vi "Plug_in_BMT_data.vi"() -> (5 "Plug in titles":string[](array[string])=["Raw data filename", "A Left", "B Left", "A Right", "B Right", "Left Bkgd", "Right Bkgd", "Left C", "Right C", "Left c'/C", "Right c'/C"], 7 "Plug in values":string[](array[string])=["18-3-99_69", "-0.030963", "0.003450", "-0.009121", "0.004121", "10.850", "6.000", "36.577", "23.514", "1.502", "1.091"])   [LabVIEW 2010]
uses:
  Globals/Meas_global.vi
  Globals/Plug_in_data_global.vi
  <vilib>/Analysis/3filter.llb/Butterworth Filter (DBL).vi
  <vilib>/Analysis/NI_AALBase.lvlib
  <vilib>/Analysis/NI_AALPro.lvlib
panel:
  in  "Smooth":bool=TRUE
  in  "Filter":bool
  out "PDF Right":cluster{"Axis":dbl[], dbl[]}(graph)={"Axis"=[-35.0, -30.0, -25.0, -20.0, -15.0, -10.0, -5.0, 0.0, 5.0, 10.0, 15.0, 20.0, 25.0, 30.0, 35.0, 40.0, 45.0, 50.0, 55.0, 60.0, 65.0, 70.0, 75.0, 80.0, 85.0, 90.0, 95.0, 100.0, 105.0, 110.0, 115.0, 120.0, 125.0, 130.0, 135.0, 140.0, 145.0, 150.0, 155.0, 160.0, 165.0, 170.0, 175.0, 180.0, 185.0, 190.0, 195.0, 200.0, 205.0, 210.0, 215.0, 220.0, 225.0, 230.0, 235.0, 240.0, 245.0, 250.0, 255.0, 260.0, 265.0, 270.0, 275.0, 280.0, 285.0, 290.0, 295.0, 300.0, 305.0, 310.0, 315.0, 320.0, 325.0, 330.0, 335.0, 340.0, 345.0, 350.0, 355.0, 360.0, 365.0, 370.0, 375.0, 380.0, 385.0, 390.0, 395.0, 400.0, 405.0, 410.0, 415.0, 420.0, 425.0, 430.0, 435.0, 440.0, 445.0, 450.0, 455.0, 460.0, 465.0, 470.0, 475.0, 480.0, 485.0, 490.0, 495.0, 500.0], [0.0, 0.0, 0.0, 6.25e-05, 0.0001875, 0.0024375, 0.0111875, 0.090375, 0.154625, 0.15925, 0.1253125, 0.0861875, 0.074625, 0.0625, 0.0445, 0.03575, 0.0279375, 0.0205, 0.0174375, 0.0135625, 0.0113125, 0.0090625, 0.0081875, 0.006625, 0.0050625, 0.005, 0.0049375, 0.003625, 0.003625, 0.003125, 0.002, 0.002375, 0.0014375, 0.0009375, 0.00125, 0.000625, 0.0005, 0.000125, 0.0005625, 0.000375, 0.000375, 0.0001875, 0.00025, 0.0003125, 0.0001875, 0.00025, 0.00025, 0.00025, 0.000125, 6.25e-05, 0.0, 0.0001875, 6.25e-05, 6.25e-05, 0.0, 0.0, 0.0, 0.0, 0.000125, 0.0, 0.0, 0.0, 0.0, 6.25e-05, 0.0, 0.0, 0.0, 0.0, 0.0, 0.0, 0.0, 0.0, 0.0, 0.0, 0.0, 0.0, 0.0, 0.0, 0.0, 0.0, 0.0, 0.0, 0.0, 0.0, 0.0, 0.0, 0.0, 0.0, 0.0, 0.0, 0.0, 0.0, 0.0, 0.0, 0.0, 0.0, 0.0, 0.0, 0.0, 0.0, 0.0, 0.0, 0.0, 6.25e-05, 0.0, 0.0, 0.0, 0.0]}
  out "PDF Left":cluster{"Axis":dbl[], dbl[]}(graph)={"Axis"=[-35.0, -30.0, -25.0, -20.0, -15.0, -10.0, -5.0, 0.0, 5.0, 10.0, 15.0, 20.0, 25.0, 30.0, 35.0, 40.0, 45.0, 50.0, 55.0, 60.0, 65.0, 70.0, 75.0, 80.0, 85.0, 90.0, 95.0, 100.0, 105.0, 110.0, 115.0, 120.0, 125.0, 130.0, 135.0, 140.0, 145.0, 150.0, 155.0, 160.0, 165.0, 170.0, 175.0, 180.0, 185.0, 190.0, 195.0, 200.0, 205.0, 210.0, 215.0, 220.0, 225.0, 230.0, 235.0, 240.0, 245.0, 250.0, 255.0, 260.0, 265.0, 270.0, 275.0, 280.0, 285.0, 290.0, 295.0, 300.0, 305.0, 310.0, 315.0, 320.0, 325.0, 330.0, 335.0, 340.0, 345.0, 350.0, 355.0, 360.0, 365.0, 370.0, 375.0, 380.0, 385.0, 390.0, 395.0, 400.0, 405.0, 410.0, 415.0, 420.0, 425.0, 430.0, 435.0, 440.0, 445.0, 450.0, 455.0, 460.0, 465.0, 470.0, 475.0, 480.0, 485.0, 490.0, 495.0, 500.0], [0.0001875, 0.00025, 0.0003125, 0.000625, 0.00225, 0.0058125, 0.0179375, 0.1063125, 0.1238125, 0.1006875, 0.0925, 0.074875, 0.0638125, 0.05425, 0.045875, 0.0419375, 0.03625, 0.02475, 0.022625, 0.02125, 0.0186875, 0.0146875, 0.013625, 0.0095, 0.0085625, 0.0083125, 0.0081875, 0.007, 0.0065625, 0.00575, 0.0041875, 0.004875, 0.0043125, 0.0045, 0.003, 0.003375, 0.003, 0.0019375, 0.002625, 0.0025625, 0.001875, 0.0015, 0.0015, 0.0015625, 0.001625, 0.0011875, 0.00125, 0.0013125, 0.0011875, 0.0005625, 0.00075, 0.00075, 0.000875, 0.0006875, 0.0003125, 0.00075, 0.0003125, 0.0005625, 0.0003125, 0.0003125, 0.000375, 0.0005625, 0.0003125, 0.000375, 0.00025, 0.00025, 0.0005625, 0.00025, 0.0001875, 0.000375, 0.0003125, 0.0003125, 0.000125, 0.000125, 0.0001875, 6.25e-05, 0.0001875, 0.000125, 0.0, 6.25e-05, 0.0001875, 0.00025, 0.000125, 0.00025, 0.000125, 6.25e-05, 0.000125, 0.000125, 0.0, 0.000125, 6.25e-05, 0.000125, 6.25e-05, 0.0001875, 0.000125, 0.000125, 6.25e-05, 6.25e-05, 0.00025, 0.0, 6.25e-05, 0.0, 0.0, 0.0, 6.25e-05, 0.0, 6.25e-05, 0.000125]}
  in  "No of bins":i32=108
  in  "Min value":dbl=-37.5 format="%.2f"
  in  "Max value":dbl=502.5 format="%.2f"
  out "Right Bkgd ppm":dbl=6.0 format="%.2f"
  out "Left Bkgd ppm":dbl=10.85 format="%.2f"
  out "Right FID Smoothed data":T1(graph)
  out "Total time":dbl=159.92000000000004 format="%.2f"
  out "Left FID Smoothed data":T1(graph)
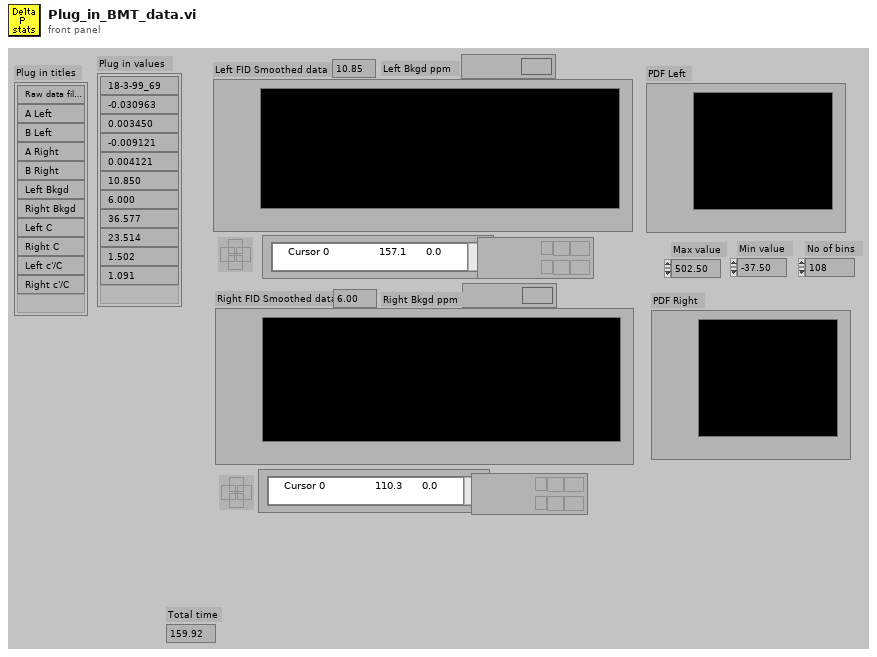
[diagram p1: front panel]
types:
  T1 = cluster{"X array Out":dbl[], "Y array Out":dbl[]}
  T2 = enum16{"Save no data", "Save data in new files", "Save data in existing files"}
  T3 = enum32{"Lowpass", "Highpass", "Bandpass", "Bandstop"}
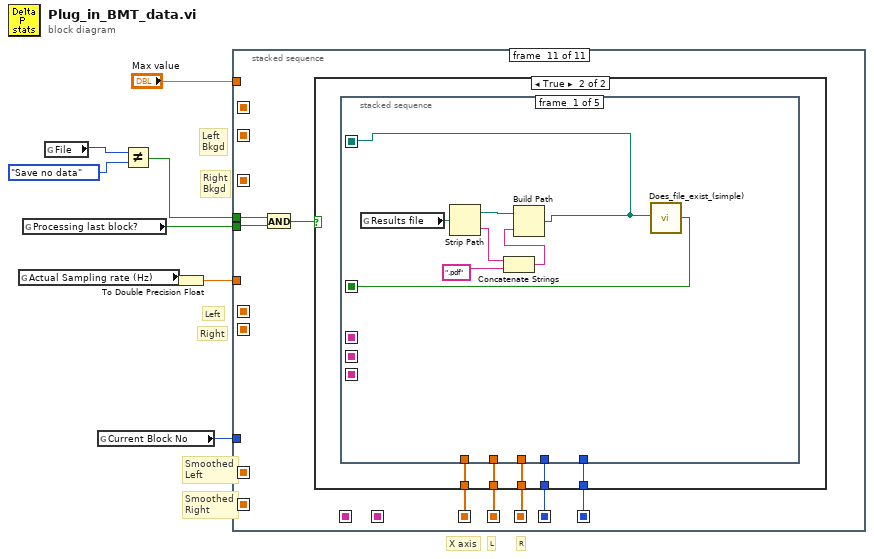
[diagram p0: block diagram]
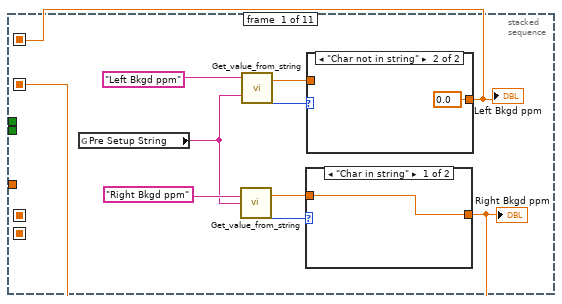
[diagram p2: hidden frame]
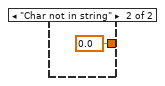
[diagram p3: hidden frame]
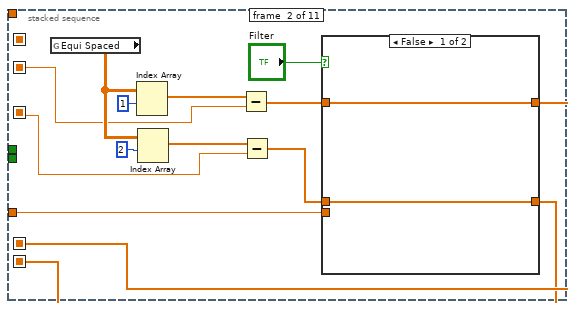
[diagram p5: hidden frame]
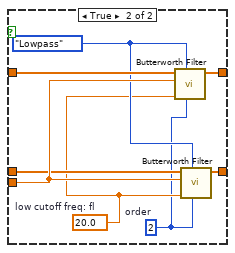
[diagram p6: hidden frame]
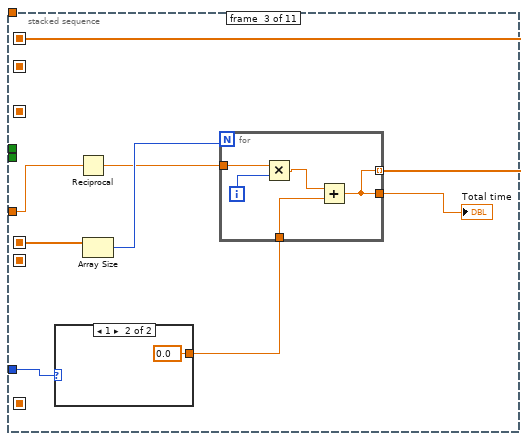
[diagram p7: hidden frame]
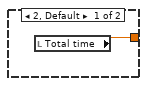
[diagram p8: hidden frame]
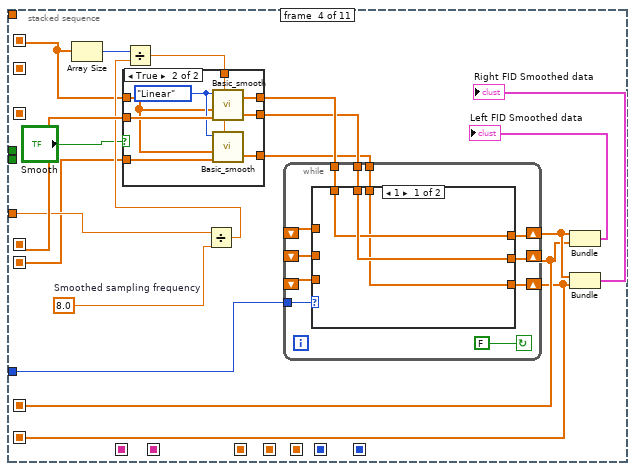
[diagram p9: hidden frame]
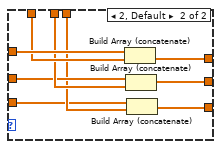
[diagram p10: hidden frame]
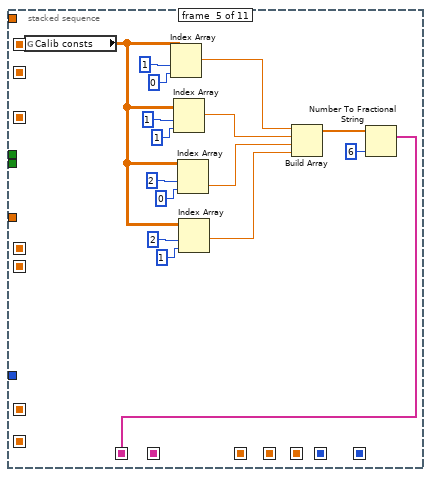
[diagram p12: hidden frame]
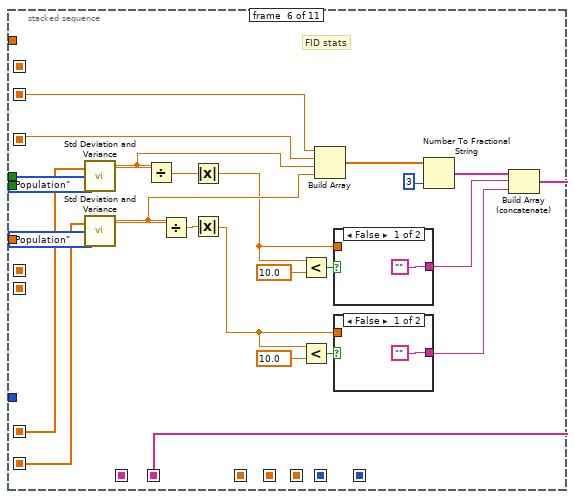
[diagram p13: hidden frame]
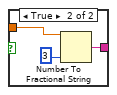
[diagram p14: hidden frame]
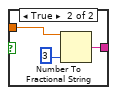
[diagram p15: hidden frame]
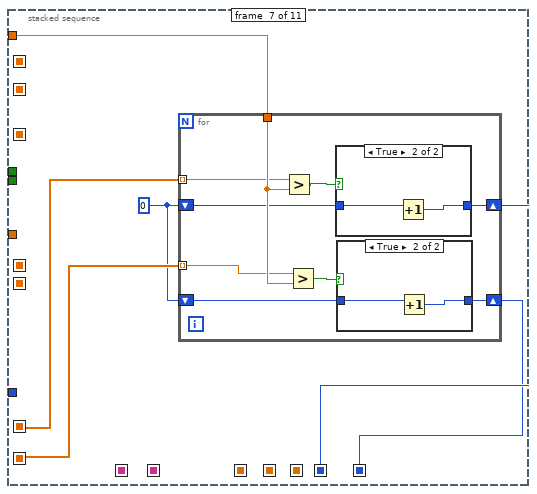
[diagram p16: hidden frame]
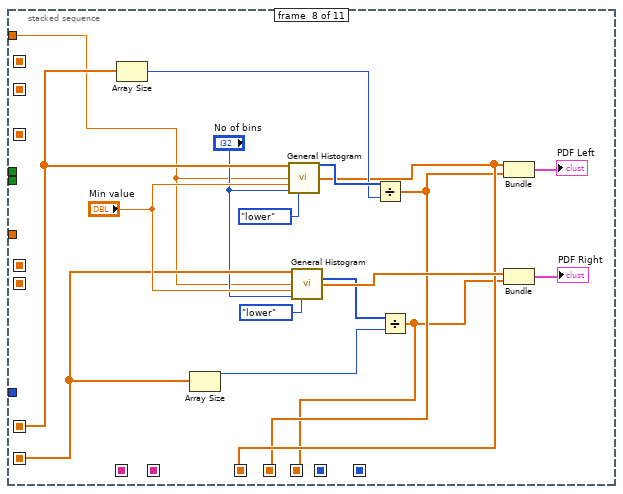
[diagram p19: hidden frame]
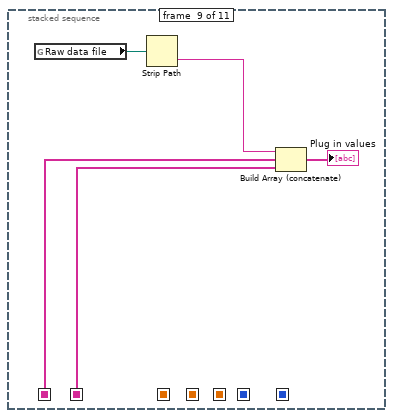
[diagram p20: hidden frame]
diagram:
  # "R"
  # "L"
  # "X axis"
  # "Smoothed\nRight"
  # "Smoothed\nLeft"
  # "Right\nBkgd"
  # "Left\nBkgd"
  # "Right"
  # "Left"
  n1 = global read "Meas_global.vi" "Actual Sampling rate (Hz)"() -> (w8:dbl)
  n2 = global read "Meas_global.vi" "Processing last block?"() -> (w5:bool)
  n3 = global read "Meas_global.vi" "File"() -> (w2:T2)
  n4 = global read "Meas_global.vi" "Current Block No"() -> (w7:i32)
  n5 = Not Equal?(x=w2, y=T2."Save no data" ("File")) -> (x != y?=w1:bool)
  n6 = To Double Precision Float(number=w8) -> (double precision float=w6:dbl)
  n7 = stacked-sequence {
    seq-local: [_ _ _ _ w112 _ _ _ _ _ _] -> [_ _ _ _ _ _ _ _ w202 _ _]
    seq-local: [_ w32 _ _ _ _ _ _ _ _ _] -> [_ _ w52 w77 _ _ _ _ _ _ _]
    seq-local: [_ _ w48 _ _ _ _ _ _ _ _] -> [_ _ _ w66 _ _ _ _ _ _ _]
    seq-local: [_ w29 _ _ _ _ _ _ _ _ _] -> [_ _ _ w67 _ _ _ _ _ _ _]
    seq-local: [w10 _ _ _ _ _ _ _ _ _ _] -> [_ w27 _ _ _ w146 _ _ _ _ _]
    seq-local: [w9 _ _ _ _ _ _ _ _ _ _] -> [_ w25 _ _ _ w145 _ _ _ _ _]
    seq-local: [_ _ _ w62 _ _ _ _ _ _ _] -> [_ _ _ _ _ w151 w164 w197 _ _ _]
    seq-local: [_ _ _ w61 _ _ _ _ _ _ _] -> [_ _ _ _ _ w149 w163 w195 _ _ _]
    seq-local: [_ _ _ _ _ w130 _ _ _ _ _] -> [_ _ _ _ _ _ _ _ w200 _ _]
    seq-local: [_ _ _ _ _ _ _ w184 _ _ _] -> [_ _ _ _ _ _ _ _ _ _ w222]
    seq-local: [_ _ _ _ _ _ _ w182 _ _ _] -> [_ _ _ _ _ _ _ _ _ _ w221]
    seq-local: [_ _ _ _ _ _ w161 _ _ _ _] -> [_ _ _ _ _ _ _ _ _ _ w220]
    seq-local: [_ _ _ _ _ _ w160 _ _ _ _] -> [_ _ _ _ _ _ _ _ _ _ w219]
    seq-local: [_ _ _ _ _ _ _ w181 _ _ _] -> [_ _ _ _ _ _ _ _ _ _ w218]
    tunnel: w6 -> [_ w30 w50 w75 _ _ _ _ _ _ _]
    tunnel: w7 -> [_ _ w45 w68 _ _ _ _ _ _ _]
    tunnel: w5 -> [_ _ _ _ _ _ _ _ _ _ w217]
    tunnel: "Max value" -> [_ _ _ _ _ _ w165 w183 _ _ _]
    tunnel: w1 -> [_ _ _ _ _ _ _ _ _ _ w216]
    frame #0 {
      n8 = global read "Meas_global.vi" "Pre Setup String"() -> (w11:string)
      n9 = call "Get_value_from_string.vi"("Input string"=w11, "Variable name"="Right Bkgd ppm") -> ("Status"=w14:enum16{"Char in string", "Char not in string"}, "Value"=w15:dbl)  [unwired: 1 in]
      n10 = call "Get_value_from_string.vi"("Input string"=w11, "Variable name"="Left Bkgd ppm") -> ("Status"=w17:enum16{"Char in string", "Char not in string"}, "Value"=w16:dbl)  [unwired: 1 in]
      n11 = case shown="\"Char in string\"" w14 {
        tunnel: [w18 0.0 ("Value")] -> w9
        tunnel: w15 -> [w18 _]
        frame "Char in string" {
        }
        frame "Char not in string" {
        }
      }
      "Right Bkgd ppm" <- w9
      n12 = case shown="\"Char not in string\"" w17 {
        tunnel: [w20 0.0 ("Value")] -> w10
        tunnel: w16 -> [w20 _]
        frame "Char in string" {
        }
        frame "Char not in string" {
        }
      }
      "Left Bkgd ppm" <- w10
    }
    frame #1 {
      n13 = global read "Plug_in_data_global.vi" "Equi Spaced"() -> (w31:dbl[][])
      n14 = Index Array(array=w31, index (row)=1) -> (element=w28:dbl[])  [unwired: 1 in]
      n15 = Index Array(array=w31, index (row)=2) -> (element=w26:dbl[])  [unwired: 1 in]
      n16 = Subtract(x=w28, y=w27) -> (x-y=w24:dbl[])
      n17 = Subtract(x=w26, y=w25) -> (x-y=w23:dbl[])
      n18 = case shown="False" "Filter" {
        tunnel: [w36 w44] -> w32
        tunnel: w30 -> [_ w43]
        tunnel: [w35 w42] -> w29
        tunnel: w24 -> [w36 w41]
        tunnel: w23 -> [w35 w40]
        frame False {
        }
        frame True {
          w38 = 20.0  # low cutoff freq: fl
          w37 = 2  # order
          w39 = T3."Lowpass" ("filter type")
          n19 = call-poly <vilib>:"Butterworth Filter.vi"("order"=w37, "filter type"=w39, "low cutoff freq: fl"=w38, "sampling freq: fs"=w43, "X"=w41) -> ("Filtered X"=w44:dbl[])  [unwired: 3 in, 1 out]
          n20 = call-poly <vilib>:"Butterworth Filter.vi"("order"=w37, "filter type"=w39, "low cutoff freq: fl"=w38, "sampling freq: fs"=w43, "X"=w40) -> ("Filtered X"=w42:dbl[])  [unwired: 3 in, 1 out]
        }
      }
    }
    frame #2 {
      n21 = case shown="1" w45 {
        tunnel: [w53 0.0 ("Total time")] -> w46
        frame 2, Default {
          n22 = local read "Total time"() -> (w53:dbl)
        }
        frame 1 {
        }
      }
      n23 = Reciprocal(x=w50) -> (1/x=w49:dbl)
      n24 = Array Size(array=w52) -> (size(s)=w51:i32)
      n25 = for {
        N: w51 -> [_]
        tunnel: w49 -> [w58]
        tunnel: [w56] -> w48 mode=indexing
        tunnel: [w56] -> w47
        tunnel: w46 -> [w55]
        i -> [w59]
        n26 = Multiply(x=w58, y=w59) -> (x*y=w57:dbl)
        n27 = Add(x=w57, y=w55) -> (x+y=w56:dbl)
      }
      "Total time" <- w47
    }
    frame #3 {
      w76 = 8.0  # Smoothed sampling frequency
      n28 = Array Size(array=w66) -> (size(s)=w74:i32)
      n29 = Divide(x=w75, y=w76) -> (x/y=w73:dbl)
      n30 = Divide(x=w74, y=w73) -> (x/y=w72:dbl)
      n31 = case shown="True" "Smooth" {
        tunnel: w77 -> [w102 w111]
        tunnel: w72 -> [_ w110]
        tunnel: [w103 w109] -> w71
        tunnel: [w102 w108] -> w70
        tunnel: w67 -> [w101 w106]
        tunnel: w66 -> [w103 w105]
        tunnel: [w101 w104] -> w65
        frame False {
        }
        frame True {
          w107 = enum16{"Linear", "Logarithmic"}."Linear" ("Smoothing")
          n32 = call "Basic_smooth.vi"("Smoothing"=w107, "X array in"=w105, "Y array in"=w111, "No of estimates output"=w110) -> ("X array Out"=w109:dbl[], "Y array Out"=w108:dbl[])  [unwired: 1 in]
          n33 = call "Basic_smooth.vi"("Smoothing"=w107, "X array in"=w105, "Y array in"=w106, "No of estimates output"=w110) -> ("Y array Out"=w104:dbl[])  [unwired: 1 in, 1 out]
        }
      }
      n34 = while {
        tunnel: w65 -> [w81]
        shift-left: _ -> [w80]
        shift-right: [w79] -> w61
        tunnel: w71 -> [w84]
        tunnel: w70 -> [w86]
        shift-left: _ -> [w82]
        shift-right: [w87] -> w62
        tunnel: w68 -> [w88]
        shift-left: _ -> [w83]
        shift-right: [w85] -> w64
        stop <- FALSE continue-if-true
        n35 = case shown="1" w88 {
          tunnel: [w91 w95] -> w87
          tunnel: w86 -> [w91 w97]
          tunnel: [w90 w98] -> w85
          tunnel: w84 -> [w90 w99]
          tunnel: w83 -> [_ w100]
          tunnel: w82 -> [_ w96]
          tunnel: w81 -> [w89 w94]
          tunnel: w80 -> [_ w93]
          tunnel: [w89 w92] -> w79
          frame 1 {
          }
          frame 2, Default {
            n36 = Build Array (concatenate)(w100, w99) -> (w98:dbl[])
            n37 = Build Array (concatenate)(w96, w97) -> (w95:dbl[])
            n38 = Build Array (concatenate)(w93, w94) -> (w92:dbl[])
          }
        }
      }
      n39 = Bundle("X array Out"=w64, "Y array Out"=w62) -> (→"Left FID Smoothed data":T1)  [unwired: 1 in]
      n40 = Bundle("X array Out"=w64, "Y array Out"=w61) -> (→"Right FID Smoothed data":T1)  [unwired: 1 in]
    }
    frame #4 {
      n41 = global read "Meas_global.vi" "Calib consts"() -> (w119:dbl[][])
      n42 = Index Array(array=w119, index (row)=1, index (col)=0) -> (element=w118:dbl)
      n43 = Index Array(array=w119, index (row)=1, index (col)=1) -> (element=w117:dbl)
      n44 = Index Array(array=w119, index (row)=2, index (col)=0) -> (element=w116:dbl)
      n45 = Index Array(array=w119, index (row)=2, index (col)=1) -> (element=w115:dbl)
      n46 = Build Array(w118, w117, w116, w115) -> (w114:dbl[])
      n47 = Number To Fractional String(number=w114, precision (6)=i16 6) -> (F-format string=w112:string[])  [unwired: 2 in]
    }
    frame #5 {
      # "FID stats"
      n48 = call <vilib>:"Std Deviation and Variance.vi"("X"=w151, "Weighting (Sample)"=enum16{"Sample", "Population"}."Population") -> ("mean"=w142:dbl, "standard deviation"=w143:dbl)  [unwired: 1 out]
      n49 = call <vilib>:"Std Deviation and Variance.vi"("X"=w149, "Weighting (Sample)"=enum16{"Sample", "Population"}."Population") -> ("mean"=w140:dbl, "standard deviation"=w141:dbl)  [unwired: 1 out]
      n50 = Divide(x=w143, y=w142) -> (x/y=w148:dbl)
      n51 = Divide(x=w141, y=w140) -> (x/y=w147:dbl)
      n52 = Absolute Value(x=w148) -> (abs(x)=w137:dbl)
      n53 = Absolute Value(x=w147) -> (abs(x)=w132:dbl)
      n54 = Less?(x=w137, y=10.0) -> (x < y?=w138:bool)
      n55 = Less?(x=w132, y=10.0) -> (x < y?=w134:bool)
      n56 = Build Array(w146, w145, w142, w140) -> (w144:dbl[])
      n57 = case shown="False" w138 {
        tunnel: w137 -> [_ w158]
        tunnel: ["" w157] -> w135
        frame False {
        }
        frame True {
          n58 = Number To Fractional String(number=w158, precision (6)=3) -> (F-format string=w157:string)  [unwired: 2 in]
        }
      }
      n59 = case shown="False" w134 {
        tunnel: w132 -> [_ w154]
        tunnel: ["" w153] -> w131
        frame False {
        }
        frame True {
          n60 = Number To Fractional String(number=w154, precision (6)=3) -> (F-format string=w153:string)  [unwired: 2 in]
        }
      }
      n61 = Number To Fractional String(number=w144, precision (6)=3) -> (F-format string=w136:string[])  [unwired: 2 in]
      n62 = Build Array (concatenate)(w136, w135, w131) -> (w130:string[])
    }
    frame #6 {
      w162 = 0
      n63 = for {
        tunnel: w165 -> [w174]
        tunnel: w164 -> [w173] mode=indexing
        tunnel: w163 -> [w172] mode=indexing
        shift-right: [w169] -> w161
        shift-left: w162 -> [w170]
        shift-right: [w166] -> w160
        shift-left: w162 -> [w167]
        n64 = Greater?(x=w173, y=w174) -> (0:w171:bool)
        n65 = Greater?(x=w172, y=w174) -> (0:w168:bool)
        n66 = case shown="True" w171 {
          tunnel: w170 -> [w178 w180]
          tunnel: [w178 w179] -> w169
          frame False {
          }
          frame True {
            n67 = Increment(x=w180) -> (x+1=w179:i32)
          }
        }
        n68 = case shown="True" w168 {
          tunnel: w167 -> [w175 w177]
          tunnel: [w175 w176] -> w166
          frame False {
          }
          frame True {
            n69 = Increment(x=w177) -> (x+1=w176:i32)
          }
        }
      }
    }
    frame #7 {
      n70 = Array Size(array=w197) -> (size(s)=w185:i32)
      n71 = Array Size(array=w195) -> (size(s)=w187:i32)
      n72 = call <vilib>:"General Histogram.vi"("X"=w197, "max"=w183, "min"="Min value", "# bins"="No of bins", "inclusion"=enum32{"lower", "upper"}."lower") -> ("Histogram"=w186:i32[], "Axis"=w184:dbl[])  [unwired: 6 in, 3 out]
      n73 = call <vilib>:"General Histogram.vi"("X"=w195, "max"=w183, "min"="Min value", "# bins"="No of bins", "inclusion"=enum32{"lower", "upper"}."lower") -> ("Histogram"=w188:i32[], "Axis"=w190:dbl[])  [unwired: 6 in, 3 out]
      n74 = Divide(x=w186, y=w185) -> (x/y=w182:dbl[])
      n75 = Divide(x=w188, y=w187) -> (x/y=w181:dbl[])
      n76 = Bundle("Axis"=w184, w182) -> (→"PDF Left":cluster{"Axis":dbl[], dbl[]})  [unwired: 1 in]
      n77 = Bundle("Axis"=w190, w181) -> (→"PDF Right":cluster{"Axis":dbl[], dbl[]})  [unwired: 1 in]
    }
    frame #8 {
      n78 = global read "Meas_global.vi" "Raw data file"() -> (w199:path)
      n79 = Strip Path(path=w199) -> (name=w198:string)  [unwired: 1 out]
      n80 = Build Array (concatenate)(w198, w202, w200) -> (→"Plug in values":string[])
    }
    frame #9 {
      n81 = Build Array("Raw data filename", "A Left", "B Left", "A Right", "B Right", "Left Bkgd", "Right Bkgd", "Left C", "Right C", "Left c'/C", "Right c'/C") -> (→"Plug in titles":string[])
    }
    frame #10 {
      n82 = And(x=w216, y=w217) -> (x .and. y?=w215:bool)
      n83 = case shown="True" w215 {
        tunnel: w222 -> [_ w227]
        tunnel: w221 -> [_ w226]
        tunnel: w220 -> [_ w225]
        tunnel: w219 -> [_ w224]
        tunnel: w218 -> [_ w223]
        frame False {
        }
        frame True {
          n84 = stacked-sequence {
            seq-local: [w228 _ _ _ _] -> [_ _ _ _ w274]
            seq-local: [w234 _ _ _ _] -> [_ w236 _ _ _]
            seq-local: [_ w235 _ _ _] -> [_ _ _ _ w277]
            seq-local: [_ _ w251 _ _] -> [_ _ _ _ w276]
            seq-local: [_ _ _ w261 _] -> [_ _ _ _ w275]
            tunnel: w227 -> [_ w237 _ _ _]
            tunnel: w226 -> [_ _ w259 _ _]
            tunnel: w225 -> [_ _ w255 _ _]
            tunnel: w224 -> [_ _ _ w265 _]
            tunnel: w223 -> [_ _ _ w266 _]
            frame #0 {
              n85 = global read "Meas_global.vi" "Results file"() -> (w233:path)
              n86 = Strip Path(path=w233) -> (stripped path=w232:path, name=w231:string)
              n87 = Concatenate Strings(w231, ".pdf" ("Results file")) -> (w229:string)
              n88 = Build Path(base path=w232, name or relative path=w229) -> (appended path=w228:path)
              n89 = call "Does_file_exist_(simple).vi"("Pathname"=w228) -> ("exists?"=w234:bool)
            }
            frame #1 {
              n90 = case shown="False" w236 {
                tunnel: w237 -> [w249 _]
                tunnel: [w240 ""] -> w235
                frame False {
                  w239 = "\r"
                  n91 = call "Date_and_Time_to_string.vi"() -> ("Date and time (spreadsheet)"=w241:string)
                  n92 = Number To Fractional String(number=w249, precision (6)=i16 3) -> (F-format string=w247:string[])  [unwired: 2 in]
                  n93 = Build Array (concatenate)("Run No", "No of Overflows", "X axis", w247) -> (w243:string[])
                  n94 = Array To Spreadsheet String(array=w243, 3:"%s" ("format string")) -> (spreadsheet string=w238:string)  [unwired: 1 in]
                  n95 = Concatenate Strings(w241, w239, w238, w239) -> (w240:string)
                }
                frame True {
                }
              }
            }
            frame #2 {
              n96 = global read "Meas_global.vi" "Comments"() -> (w257:string)
              n97 = Number To Decimal String(number=w255) -> (decimal integer string=w256:string)  [unwired: 1 in]
              n98 = Number To Fractional String(number=w259, precision (6)=i16 6) -> (F-format string=w258:string[])  [unwired: 2 in]
              n99 = Build Array (concatenate)(w257, w256, "Left" ("Comments"), w258) -> (w252:string[])
              n100 = Array To Spreadsheet String(array=w252, 3:"%s" ("format string")) -> (spreadsheet string=w251:string)  [unwired: 1 in]
            }
            frame #3 {
              n101 = Number To Decimal String(number=w265) -> (decimal integer string=w269:string)  [unwired: 1 in]
              n102 = Number To Fractional String(number=w266, precision (6)=i16 6) -> (F-format string=w264:string[])  [unwired: 2 in]
              n103 = Build Array (concatenate)("", w269, "Right" ("Comments"), w264) -> (w262:string[])
              n104 = Array To Spreadsheet String(array=w262, 3:"%s" ("format string")) -> (spreadsheet string=w261:string)  [unwired: 1 in]
            }
            frame #4 {
              w272 = TRUE  # append to file? (new file:F)
              n105 = Concatenate Strings(w277, w276, w275, "\r") -> (w273:string)
              n106 = call "Write_Characters_To_File.vi"("file path (dialog if empty)"=w274, "character string"=w273, "append to file? (new file:F)"=w272) -> ()  [unwired: 5 in, 1 out]
            }
          }
        }
      }
    }
  }
